vi "Destroy.vi"(8 "error in (no error)":errorcluster, 11 "Cluster In":refnum<class "Cluster.lvclass">) -> (0 "error out":errorcluster, 3 "Cluster Out":refnum<class "Cluster.lvclass">)   [LabVIEW 2017, in "Front Panel Publisher.lvlib" / "Cluster.lvclass"]
uses:
  Cluster.lvclass
  Object_class/Object.lvclass
  Control_class/Control.lvclass
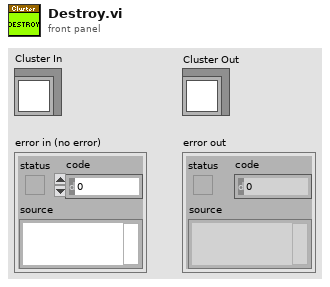
[diagram p1: front panel]
types:
  T1 = typedef "Front Panel Publisher.lvlib/Cluster.lvclass/Attributes.ctl" = cluster{"Cluster Decoration":refnum<class "Object.lvclass">, "Cluster Objects":refnum<class "Object.lvclass">[]}
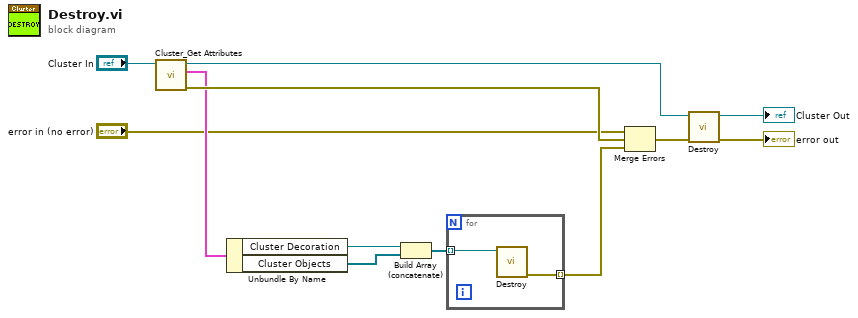
[diagram p0: block diagram]
diagram:
  n1 = call "Cluster_Get Attributes.vi"("Cluster In"="Cluster In") -> ("error out"=w7:errorcluster, "Cluster Attributes"=w6:T1, "Cluster Out"=w11:refnum<class "Cluster.lvclass">)  [unwired: 8 in]
  n2 = Unbundle By Name(w6) -> ("Cluster Decoration"=w5:refnum<class "Object.lvclass">, "Cluster Objects"=w4:refnum<class "Object.lvclass">[])
  n3 = Build Array (concatenate)(w5, w4) -> (w3:refnum<class "Object.lvclass">[])
  n4 = for {
    tunnel: w3 -> [w14] mode=indexing
    tunnel: [w13] -> w1 mode=indexing
    n5 = call-dynamic "Destroy.vi"("Object In"=w14) -> ("error out"=w13:errorcluster)  [unwired: 9 in, 1 out]
  }
  n6 = Merge Errors("error in (no error)", w7, w1) -> (w8:errorcluster)
  n7 = call-parent "Destroy.vi"("error in (no error)"=w8, "Control In"=w11) -> ("error out"=→"error out":errorcluster, "Control Out"=→"Cluster Out":refnum<class "Cluster.lvclass">)  [unwired: 8 in]
